vi "ReadBridge.vi"() -> ()   [LabVIEW 2015]
panel:
  in  "error in (no error)":errorcluster
  out "error out":errorcluster
  out "String 4":string
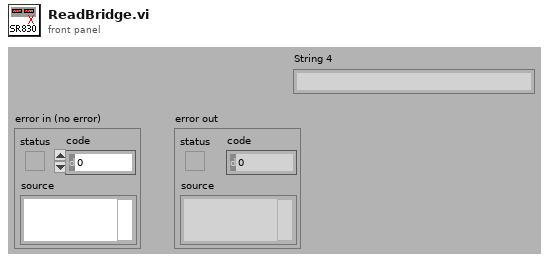
[diagram p1: front panel]
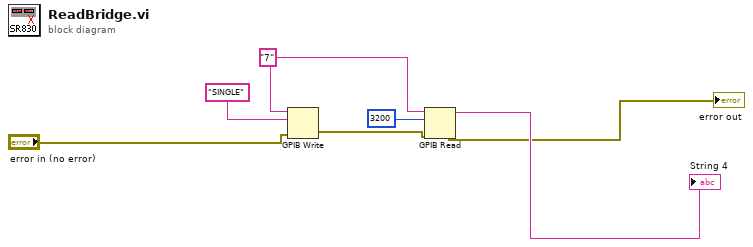
[diagram p0: block diagram]
diagram:
  w2 = "7"
  n1 = GPIB Write(0:w2, 1:"SINGLE", 3:"error in (no error)") -> (6:w7:errorcluster)  [unwired: 2 in, 1 out]
  n2 = GPIB Read(0:w2, 1:3200, 3:w7) -> (5:→"String 4":string, 7:→"error out":errorcluster)  [unwired: 2 in, 1 out]
